vi "Get Default Pressure Units.vi"(8 "error in (no error)":errorcluster, 11 "VISA resource name":refnum<visa-resource-name>) -> (0 "error out":errorcluster, 2 "Default Pressure Units":i32, 3 "VISA resource name out":refnum<visa-resource-name>)   [LabVIEW 2014, in "Fluke 5XXX Series Multicalibrators.lvlib"]
doc: "This VI returns the power-up and reset default pressure display units.\n\nNote:\n\nThis VI is available only for instrument model 5520A with option 700P (pressure modules)."
uses:
  Fluke 5XXX Series Multicalibrators.lvlib
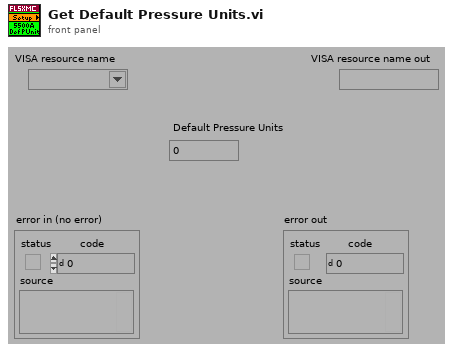
[diagram p1: front panel]
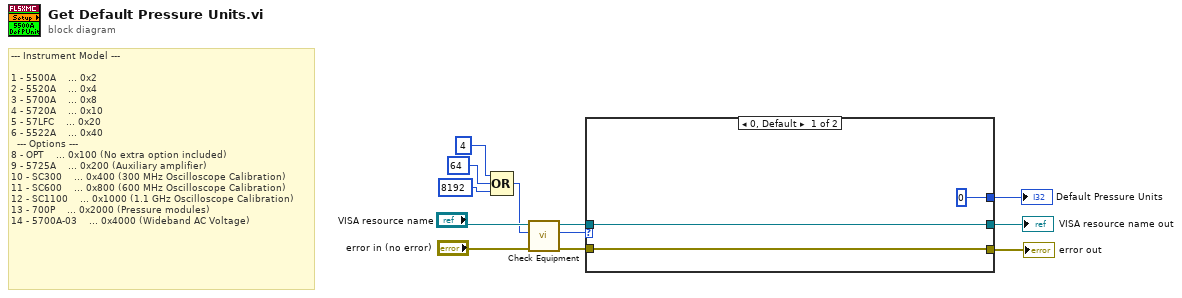
[diagram p0: block diagram]
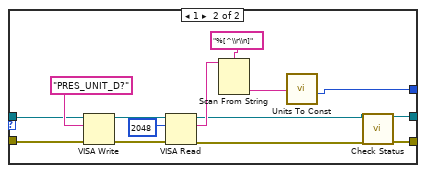
[diagram p2: hidden frame]
diagram:
  # "--- Instrument Model ---\n\n1 - 5500A    ... 0x2\n2 - 5520A    ... 0x4\n3 - 5700A    ... 0x8\n4 - 5720A    ... 0x10\n5 - 57LFC    ... 0x20\n6 - 5522A    ... 0x40\n  --- Options ---\n8 - OPT    ... 0x100 (No extra option included)\n9 - 5725A    ... 0x200 (Auxiliary amplifier)\n10 - SC300    ... 0x400 (300 MHz Oscilloscope Calibration)\n11 - SC600    ... 0x800 (600 MHz Oscilloscope Calibration)\n12 - SC1100    ... 0x1000 (1.1 GHz Oscilloscope Calibration)\n13 - 700P    ... 0x2000 (Pressure modules)\n14 - 5700A-03    ... 0x4000 (Wideband AC Voltage)"
  n1 = Compound Arithmetic op=OR(4 ("Numeric"), 64 ("Numeric"), 8192 ("Numeric")) -> (w3:i32)
  n2 = call "Check Equipment.vi"("error in (no error)"="error in (no error)", "Bit Mask"=w3, "VISA resource name"="VISA resource name") -> ("error out"=w12:errorcluster, "Present?"=w11:u32, "VISA resource name out"=w10:refnum<visa-resource-name>)  [unwired: 6 in]
  n3 = case shown="0, Default" w11 {
    tunnel: [w15 w23] -> w7
    tunnel: [w14 w22] -> w6
    tunnel: w12 -> [w15 w25]
    tunnel: w10 -> [w14 w24]
    tunnel: [0 w19] -> w2
    frame 0, Default {
    }
    frame 1 {
      n4 = VISA Write(VISA resource name=w24, write buffer="PRES_UNIT_D?", error in (no error)=w25) -> (VISA resource name out=w28:refnum<visa-resource-name>, error out=w27:errorcluster)  [unwired: 1 out]
      n5 = VISA Read(VISA resource name=w28, byte count=u32 2048 ("byte count (0)"), error in (no error)=w27) -> (VISA resource name out=w17:refnum<visa-resource-name>, read buffer=w20:string, error out=w18:errorcluster)  [unwired: 1 out]
      n6 = Scan From String(format string="%[^\\r\\n]", input string=w20) -> (output 1=w16:string)  [unwired: 3 in, 3 out]
      n7 = call "Units To Const.vi"("Units"=w16) -> ("Const"=w19:i32)  [unwired: 10 in]
      n8 = call "Check Status.vi"("VISA resource name"=w17, "error in (no error)"=w18) -> ("VISA resource name out"=w22:refnum<visa-resource-name>, "error out"=w23:errorcluster)  [unwired: 12 in]
    }
  }
  "Default Pressure Units" <- w2
  "VISA resource name out" <- w6
  "error out" <- w7
